vi "GEOM_VAR_BinCorrectedFPA.vi"(9 "Action":T1, 10 "GEOM_BinCorrectedFPA in":T2[](array[typedef])) -> (2 "GEOM_BinCorrectedFPA out":T2[](array[typedef]))   [LabVIEW 2016]
uses:
  GEOM_CorrectedFPA.ctl
  GEOM_VAR_action.ctl
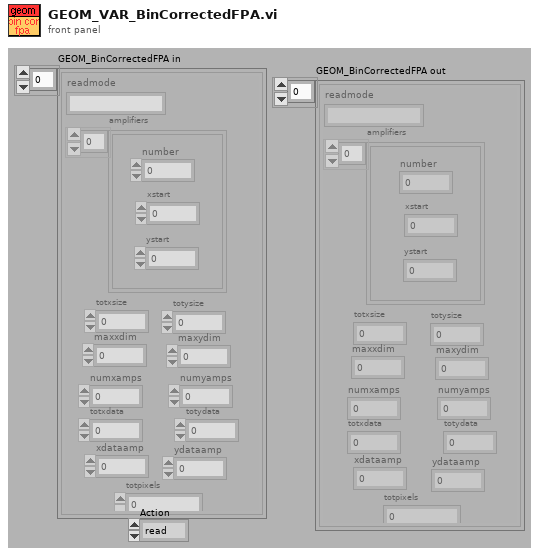
[diagram p1: front panel]
types:
  T1 = typedef "GEOM_VAR_action.ctl" = enum16{"read", "write"}
  T2 = typedef "GEOM_CorrectedFPA.ctl" = cluster{"readmode":string, "amplifiers":cluster{"number":i32, "xstart":i32, "ystart":i32}[], "totxsize":i32, "totysize":i32, "maxxdim":i32, "maxydim":i32, "numxamps":i32, "numyamps":i32, "totxdata":i32, "totydata":i32, "xdataamp":i32, "ydataamp":i32, "totpixels":i32}
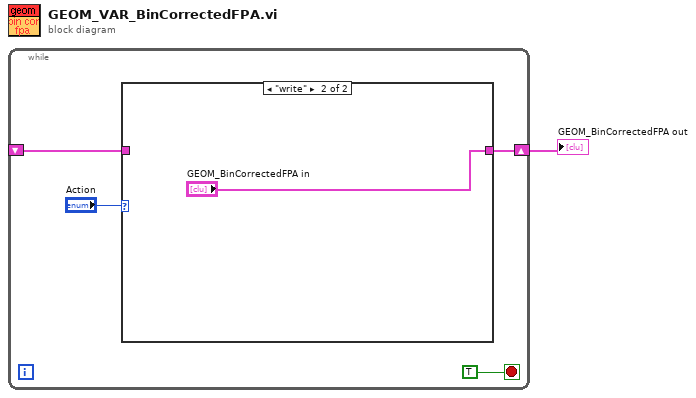
[diagram p0: block diagram]
diagram:
  n1 = while {
    shift-right: [w4] -> w1
    shift-left: _ -> [w3]
    stop <- TRUE stop-if-true
    n2 = case shown="\"write\"" "Action" {
      tunnel: [w6 "GEOM_BinCorrectedFPA in"] -> w4
      tunnel: w3 -> [w6 _]
      frame "read", Default {
      }
      frame "write" {
      }
    }
  }
  "GEOM_BinCorrectedFPA out" <- w1
